vi "Move Window.vi"(8 "error in (no error)":errorcluster, 10 "window position":cluster{"Left":i16, "Top":i16}, 11 "VI Ref":refnum<vi>) -> (0 "error out":errorcluster)   [LabVIEW 2017, in "DSF Core.lvlib" / "Thread.lvclass"]
uses:
  Thread.lvclass
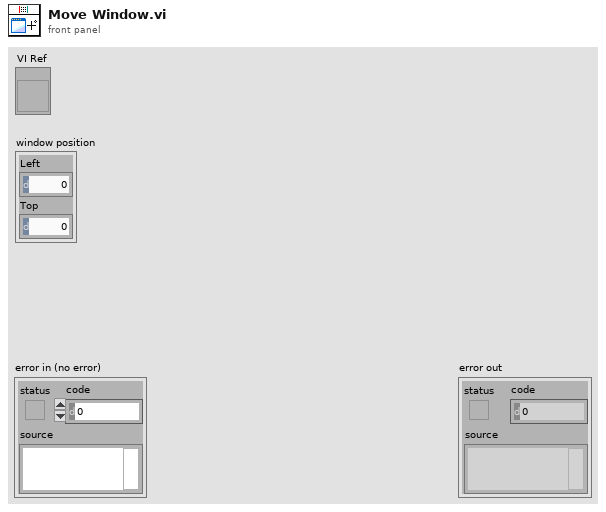
[diagram p1: front panel]
types:
  T1 = typedef "LVRectTypeDef.ctl" = cluster{"Left":i16, "Top":i16, "Right":i16, "Bottom":i16}
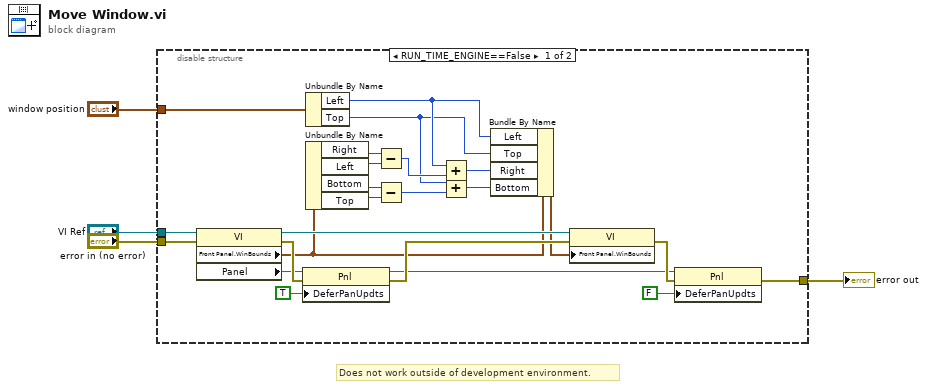
[diagram p0: block diagram]
diagram:
  # "Does not work outside of development environment."
  n1 = disable-structure shown="RUN_TIME_ENGINE==False" {
    disable-tunnel: "error in (no error)" -> [w12 w29]
    disable-tunnel: "window position" -> [w11 _]
    disable-tunnel: "VI Ref" -> [w10 _]
    disable-tunnel: [w9 w29] -> w1
    frame condition #0 (active) {
      n2 = property class="VI"(reference=w10, error in=w12) -> (reference out=w7:refnum<vi>, error out=w16:errorcluster, "Front Panel.WinBounds"=w5:T1, "Panel"=w8:refnum<vi>)
      n3 = property class="Pnl"(reference=w8, error in=w16, "DeferPanUpdts"=TRUE ("Defer Panel Updates")) -> (reference out=w13:refnum<vi>, error out=w28:errorcluster)
      n4 = Unbundle By Name(w11) -> ("Left"=w23:i16, "Top"=w20:i16)
      n5 = Unbundle By Name(w5) -> ("Right"=w27:i16, "Left"=w26:i16, "Bottom"=w25:i16, "Top"=w24:i16)
      n6 = Subtract(x=w27, y=w26) -> (x-y=w21:i16)
      n7 = Subtract(x=w25, y=w24) -> (x-y=w18:i16)
      n8 = Add(x=w23, y=w21) -> (x+y=w22:i16)
      n9 = Add(x=w20, y=w18) -> (x+y=w19:i16)
      n10 = Bundle By Name(cluster=w5, "Left"=w23, "Top"=w20, "Right"=w22, "Bottom"=w19) -> (w6:T1)
      n11 = property class="VI"(reference=w7, error in=w28, "Front Panel.WinBounds"=w6) -> (error out=w14:errorcluster)  [unwired: 1 out]
      n12 = property class="Pnl"(reference=w13, error in=w14, "DeferPanUpdts"=FALSE ("Defer Panel Updates")) -> (error out=w9:errorcluster)  [unwired: 1 out]
    }
    frame condition #1 {
    }
  }
  "error out" <- w1
